vi "mqttCmdAcknowledge.vi"(0 "_mqtt in":refnum<class "mqttCmdPublish.lvclass">, 7 "mqtt in":refnum<class "mqtt.lvclass">, 11 "error in (no error)":errorcluster) -> (4 "_mqtt out":refnum<class "mqttCmdPublish.lvclass">, 8 "notification":T1, 15 "error out":errorcluster)   [LabVIEW 2014, in "labview-mqtt.lvlib" / "mqttCmdPublish.lvclass"]
uses:
  mqttCmdPublish.lvclass
  mqttTypedef/mqttRXdataCluster.ctl
  mqttTypedef/mqttFixedHeaderResponse.ctl
  mqttTypedef/mqttQOSlevel.ctl
  mqttTypedef/mqttMessageType.ctl
  mqtt.lvclass
  mqttCmd.lvclass/mqttCmd.ctl
  labview-mqtt.lvlib
  mqttCmd.lvclass
panel:
  out "timed out? 2":bool
  out "timed out?":bool
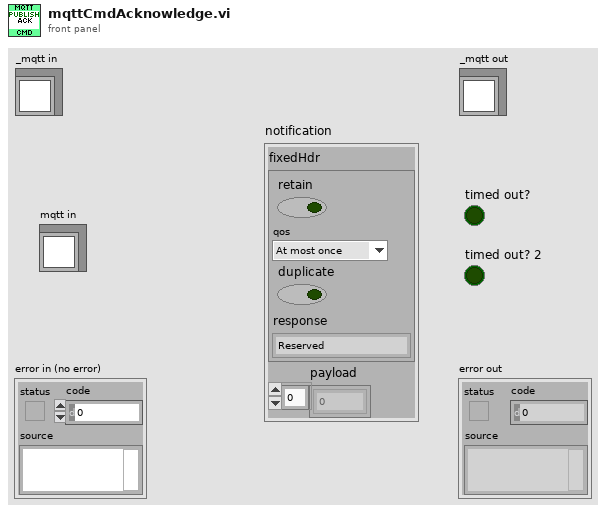
[diagram p1: front panel]
types:
  T1 = typedef "labview-mqtt.lvlib/mqttRXdataCluster.ctl" = cluster{"fixedHdr":T2, "payload":u8[]}
  T2 = typedef "labview-mqtt.lvlib/mqttFixedHeaderResponse.ctl" = cluster{"retain":bool, "qos":T3, "duplicate":bool, "response":T4}
  T3 = typedef "labview-mqtt.lvlib/mqttQOSlevel.ctl" = enum8{"At most once", "At least once", "Exactly once", "Reserved"}
  T4 = typedef "labview-mqtt.lvlib/mqttMessageType.ctl" = enum32{"Reserved", "CONNECT", "CONNACK", "PUBLISH", "PUBACK", "PUBREC", "PUBREL", "PUBCOMP", "SUBSCRIBE", "SUBACK", "UNSUBSCRIBE", "UNSUBACK", "PINGREQ", "PINGRESP", "DISCONNECT", "Reserved2"}
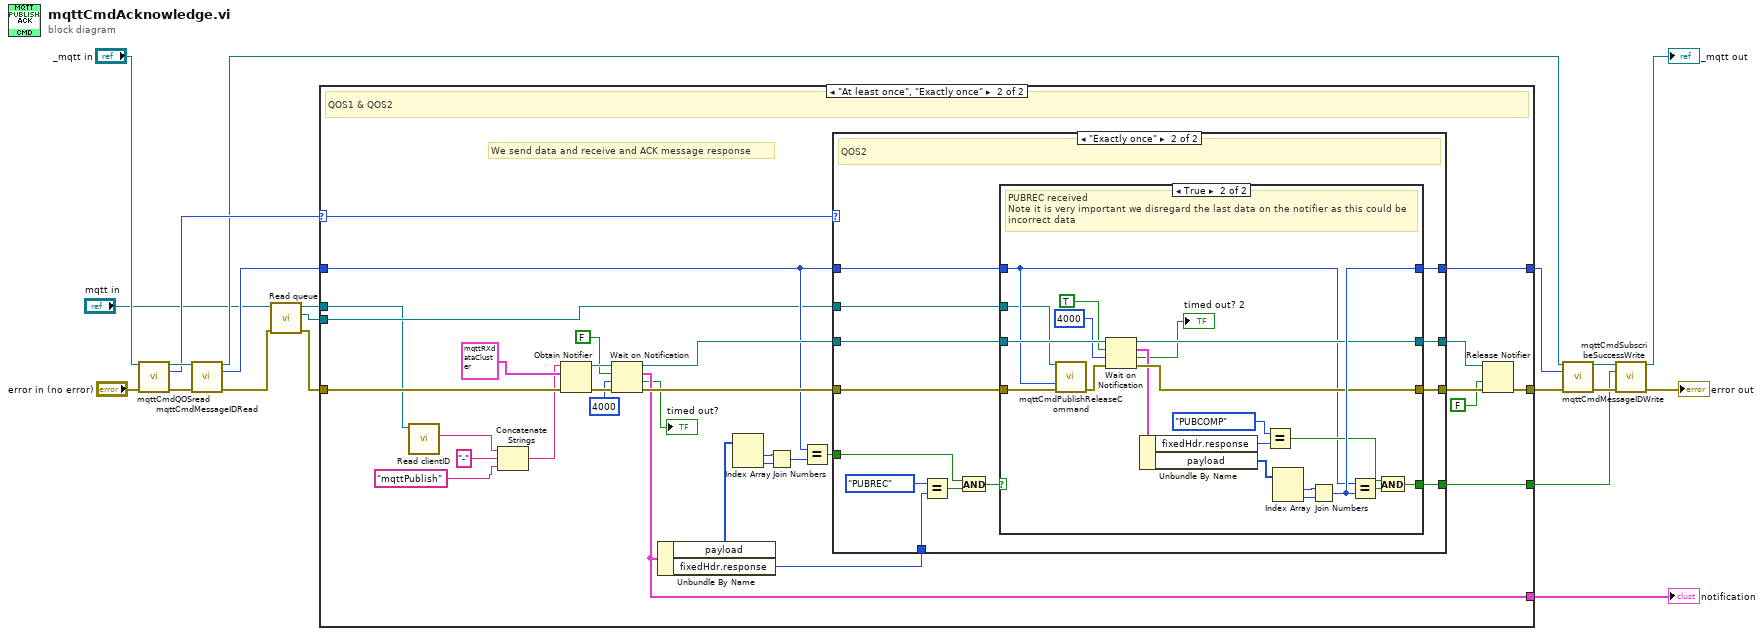
[diagram p0: block diagram]
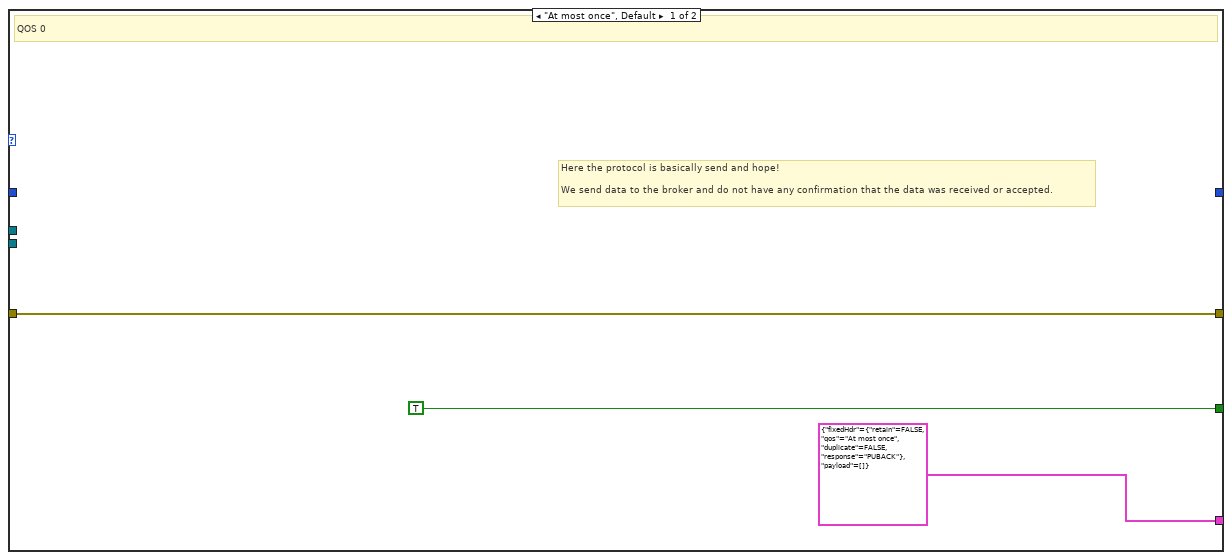
[diagram p2: hidden frame]
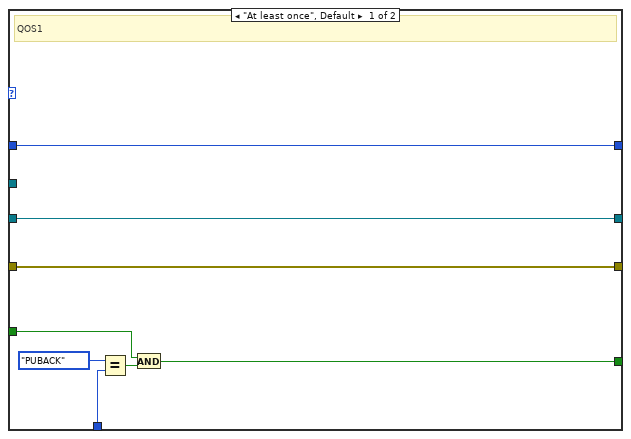
[diagram p3: hidden frame]
diagram:
  n1 = call "mqttCmdQOSread.vi"("mqttBrokerCommand in"="_mqtt in", "error in (no error)"="error in (no error)") -> ("mqttBrokerCommand out"=w18:refnum<class "mqttCmdPublish.lvclass">, "QoS"=w16:T3, "error out"=w19:errorcluster)  [unwired: 11 in]
  n2 = call "mqttCmdMessageIDRead.vi"("mqttBrokerCommand in"=w18, "error in (no error)"=w19) -> ("mqttBrokerCommand out"=w6:refnum<class "mqttCmdPublish.lvclass">, "messageID"=w17:u16, "error out"=w3:errorcluster)  [unwired: 11 in]
  n3 = call-dynamic "Read queue.vi"("error in (no error)"=w3, "mqtt in"="mqtt in") -> ("error out"=w2:errorcluster, "queue"=w4:refnum<queue>, "mqtt out"=w1:refnum<class "mqtt.lvclass">)  [unwired: 7 in]
  n4 = case shown="\"At least once\", \"Exactly once\"" w16 {
    selector: w16 -> [_ w53]
    tunnel: [w23 w41] -> w14
    tunnel: w2 -> [w23 w48]
    tunnel: [_ w51] -> w13
    tunnel: [TRUE w52] -> w8
    tunnel: w17 -> [_ w35]
    tunnel: [T1 {"fixedHdr"={"retain"=FALSE, "qos"=enum."At most once", "duplicate"=FALSE, "response"=enum."PUBACK"}, "payload"=[]} ("notification") w32] -> w15
    tunnel: w4 -> [_ w29]
    tunnel: w1 -> [_ w26]
    frame "At most once", Default {
      # "Here the protocol is basically send and hope!\n\nWe send data to the broker and do not have any confirmation that the data was received or accepted."
      # "QOS 0"
    }
    frame "At least once", "Exactly once" {
      # "We send data and receive and ACK message response"
      # "QOS1 & QOS2"
      n5 = call-dynamic "Read clientID.vi"("mqtt in"=w26) -> ("clientID"=w27:string)  [unwired: 8 in, 2 out]
      n6 = Concatenate Strings(w27, "-" ("string"), "mqttPublish" ("name (unnamed)")) -> (w24:string)
      n7 = Obtain Notifier(name (unnamed)=w24, notification data type=T1 {"fixedHdr"={"retain"=FALSE, "qos"=enum."At most once", "duplicate"=FALSE, "response"=enum."Reserved"}, "payload"=[]} ("notification"), error in (no error)=w48) -> (notifier out=w46:refnum<notifier>, error out=w50:errorcluster)  [unwired: 1 in, 1 out]
      n8 = Wait on Notification(notifier=w46, ignore previous (F)=FALSE, timeout in ms (-1)=4000, error in (no error)=w50) -> (notifier out=w45:refnum<notifier>, notification=w32:T1, timed out?=→"timed out?":bool, error out=w47:errorcluster)
      n9 = Unbundle By Name(w32) -> ("payload"=w37:u8[], "fixedHdr.response"=w33:T4)
      n10 = Index Array(array=w37) -> (element #1=w38:u8, element #2=w39:u8)  [unwired: 2 in]
      n11 = Join Numbers(hi=w38, lo=w39) -> ((hi.lo)=w36:u16)
      n12 = Equal?(x=w35, y=w36) -> (x = y?=w34:bool)
      n13 = case shown="\"Exactly once\"" w53 {
        tunnel: [w54 w72] -> w52
        tunnel: [w61 w74] -> w43
        tunnel: w47 -> [w61 w73]
        tunnel: w35 -> [w57 w64]
        tunnel: [w57 w71] -> w51
        tunnel: w33 -> [w59 w69]
        tunnel: w45 -> [w58 w68]
        tunnel: [w58 w65] -> w44
        tunnel: w34 -> [w56 w63]
        tunnel: w29 -> [_ w62]
        frame "At least once", Default {
          # "QOS1"
          n14 = Equal?(x=mqttMessageType."PUBACK", y=w59) -> (x = y?=w55:bool)
          n15 = And(x=w56, y=w55) -> (x .and. y?=w54:bool)
        }
        frame "Exactly once" {
          # "QOS2"
          n16 = Equal?(x=mqttMessageType."PUBREC", y=w69) -> (x = y?=w67:bool)
          n17 = And(x=w63, y=w67) -> (x .and. y?=w66:bool)
          n18 = case shown="True" w66 {
            selector: w66 -> [w78 _]
            tunnel: [w77 w95] -> w74
            tunnel: w73 -> [w77 w82]
            tunnel: [w78 w98] -> w72
            tunnel: w64 -> [w76 w81]
            tunnel: [w76 w97] -> w71
            tunnel: w68 -> [w75 w96]
            tunnel: [w75 w94] -> w65
            tunnel: w62 -> [_ w79]
            frame False {
            }
            frame True {
              # "PUBREC received\nNote it is very important we disregard the last data on the notifier as this could be incorrect data"
              n19 = call "mqttCmdPublishReleaseCommand.vi"("queue"=w79, "messageID"=w81, "error in (no error)"=w82) -> ("error out"=w80:errorcluster)  [unwired: 12 in]
              n20 = Wait on Notification(notifier=w96, ignore previous (F)=TRUE, timeout in ms (-1)=4000, error in (no error)=w80) -> (notifier out=w94:refnum<notifier>, notification=w90:T1, timed out?=→"timed out? 2":bool, error out=w95:errorcluster)
              n21 = Unbundle By Name(w90) -> ("fixedHdr.response"=w88:T4, "payload"=w89:u8[])
              n22 = Equal?(x=mqttMessageType."PUBCOMP", y=w88) -> (x = y?=w86:bool)
              n23 = Index Array(array=w89) -> (element #1=w92:u8, element #2=w93:u8)  [unwired: 2 in]
              n24 = Join Numbers(hi=w92, lo=w93) -> ((hi.lo)=w97:u16)
              n25 = Equal?(x=w81, y=w97) -> (x = y?=w85:bool)
              n26 = And(x=w86, y=w85) -> (x .and. y?=w98:bool)
            }
          }
        }
      }
      n27 = Release Notifier(notifier=w44, force destroy? (F)=FALSE, error in (no error)=w43) -> (error out=w41:errorcluster)  [unwired: 2 out]
    }
  }
  "notification" <- w15
  n28 = call "mqttCmdMessageIDWrite.vi"("mqttBrokerCommand in"=w6, "messageID"=w13, "error in (no error)"=w14) -> ("mqttBrokerCommand out"=w9:refnum<class "mqttCmdPublish.lvclass">, "error out"=w11:errorcluster)  [unwired: 11 in]
  n29 = call "mqttCmdSubscribeSuccessWrite.vi"("mqttBrokerCommand in"=w9, "success"=w8, "error in (no error)"=w11) -> ("mqttBrokerCommand out"=→"_mqtt out":refnum<class "mqttCmdPublish.lvclass">, "error out"=→"error out":errorcluster)  [unwired: 11 in]
